vi "CarWashServer.vi"   [LabVIEW 2024]
uses:
  <vilib>/Utility/file.llb/Write Delimited Spreadsheet (string).vi
panel:
  # "Server"
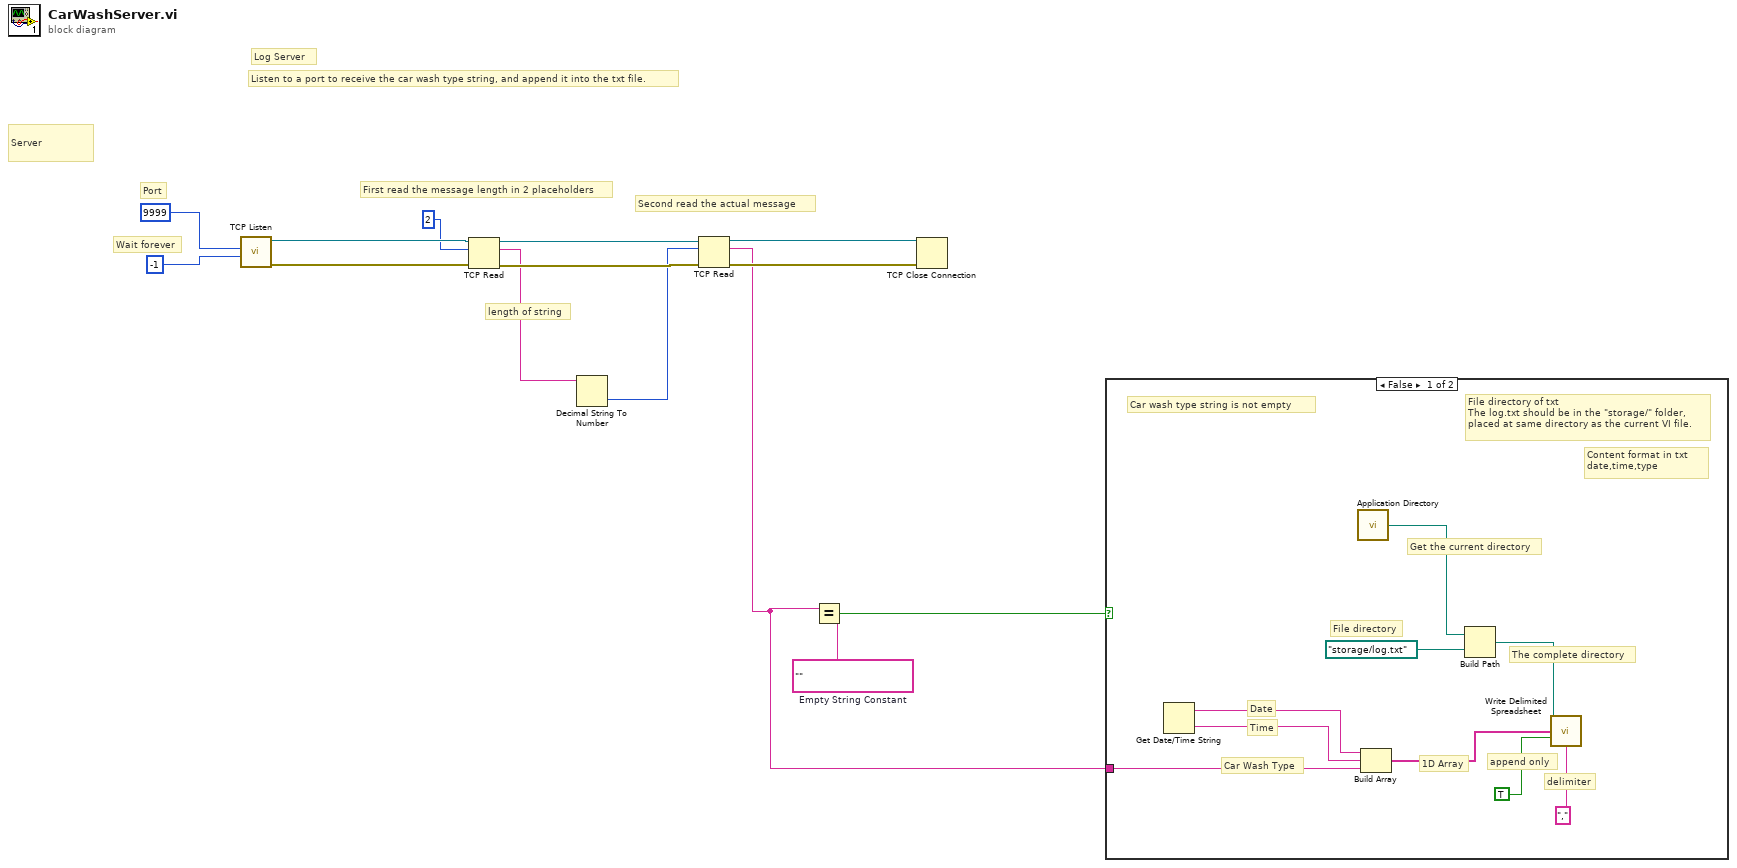
[diagram p0: block diagram]
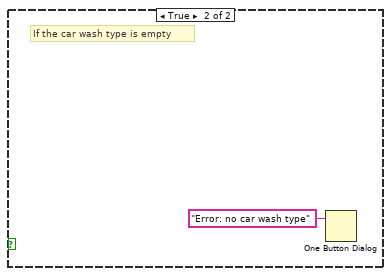
[diagram p2: hidden frame]
diagram:
  w3 = ""  # Empty String Constant
  # "Second read the actual message"
  # "First read the message length in 2 placeholders"
  # "length of string"
  # "Listen to a port to receive the car wash type string, and append it into the txt file."
  # "Log Server"
  # "Wait forever"
  # "Port"
  # "Server"
  n1 = call <vilib>:"TCP Listen.vi"("timeout ms (wait forever: -1)"=-1, "port"=u16 9999) -> ("error out"=w9:errorcluster, "connection ID"=w12:refnum<k5>)  [unwired: 5 in, 3 out]
  n2 = TCP Read(connection ID=w12, bytes to read=2, error in (no error)=w9) -> (connection ID out=w11:refnum<k5>, data out=w5:string, error out=w8:errorcluster)  [unwired: 2 in]
  n3 = Decimal String To Number(string=w5) -> (number=w4:i32)  [unwired: 2 in, 1 out]
  n4 = TCP Read(connection ID=w11, bytes to read=w4, error in (no error)=w8) -> (connection ID out=w10:refnum<k5>, data out=w1:string, error out=w7:errorcluster)  [unwired: 2 in]
  n5 = Equal?(x=w1, y=w3) -> (x = y?=w2:bool)
  n6 = TCP Close Connection(connection ID=w10, error in (no error)=w7) -> ()  [unwired: 1 in, 2 out]
  n7 = case shown="False" w2 {
    tunnel: w1 -> [w15 _]
    frame False {
      # "Car Wash Type"
      # "Car wash type string is not empty"
      # "File directory of txt\nThe log.txt should be in the \"storage/\" folder, \nplaced at same directory as the current VI file."
      # "1D Array"
      # "append only"
      # "Content format in txt\ndate,time,type"
      # "Time"
      # "Date"
      # "delimiter"
      # "The complete directory"
      # "File directory"
      # "Get the current directory"
      n8 = Get Date/Time String() -> (date string=w21:string, time string=w22:string)  [unwired: 3 in]
      n9 = call <vilib>:"Application Directory.vi"() -> ("Application Directory"=w23:path)
      n10 = Build Array "Build Array"(w21, w22, w15) -> (w20:string[])
      n11 = Build Path(base path=w23, name or relative path=path "storage/log.txt") -> (appended path=w19:path)
      n12 = call-poly <vilib>:"Write Delimited Spreadsheet.vi"("file path (dialog if empty)"=w19, "1D data"=w20, "append to file? (new file:F)"=TRUE, "delimiter (\\t)"="," ("delimiter (\\t)")) -> ()  [unwired: 10 in, 2 out]
    }
    frame True {
      # "If the car wash type is empty"
      n13 = One Button Dialog(message="Error: no car wash type") -> ()  [unwired: 1 in, 1 out]
    }
  }
